vi "Subtask 3.vi"() -> ()   [LabVIEW 2016, in "LEGO-PMR.lvrbt"]
uses:
  LEGO-PMR.lvrbt
  <vilib>/NXT/Block Support/NXT_InputPort.ctl
  <vilib>/NXT/Block Support/NXT_OutputPort.ctl
  <vilib>/NXT/Dual Mode Library/Sensors/EV3_Ultrasonic_CM.vi
  <vilib>/NXT/NXTIO Xnodes/NXTIONodeSubVIs/NXTStopMotors.vi
  <vilib>/NXT/Dual Mode Library/Display/drawText.vi
  <vilib>/NXT/Dual Mode Library/Sensors/EV3_Color_Reflect.vi
  <vilib>/NXT/Dual Mode Library/Waits/Wait_Num(msec).vi
  <vilib>/NXT/NXTIO Xnodes/NXTIONodeSubVIs/NXTMoveMotors.vi
  <vilib>/NXT/Subs/LVHSConnector.ctl
  <vilib>/NXT/NXTIO Xnodes/AddressXNode/NXTIOAddress.xnode
  <vilib>/NXT/NXTIO Xnodes/NXTIOXNode/NXTIO.xnode
  <vilib>/NXT/LegoClasses/BrickReference/BrickReference.lvclass
panel:
  out "Arm Is Up":bool
  out "Output":string
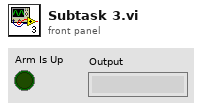
[diagram p1: front panel]
types:
  T1 = typedef "NXT_OutputPort.ctl" = u8
  T2 = typedef "NXT_InputPort.ctl" = u32
  T3 = typedef "LVHSConnector.ctl" = refnum<class "BrickReference.lvclass">
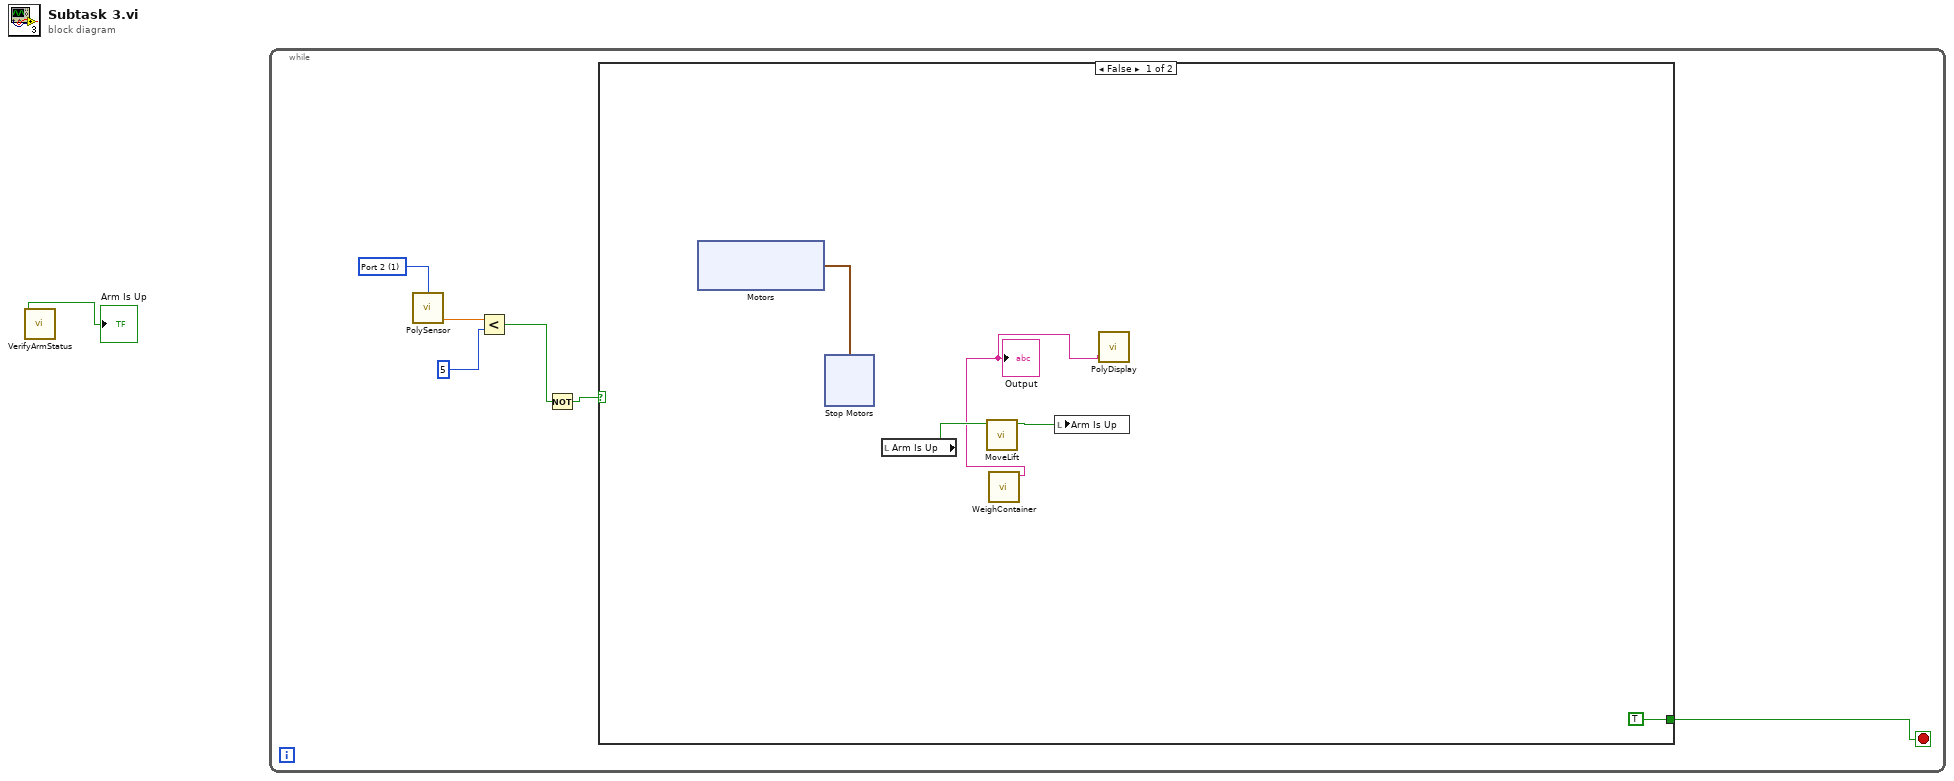
[diagram p0: block diagram]
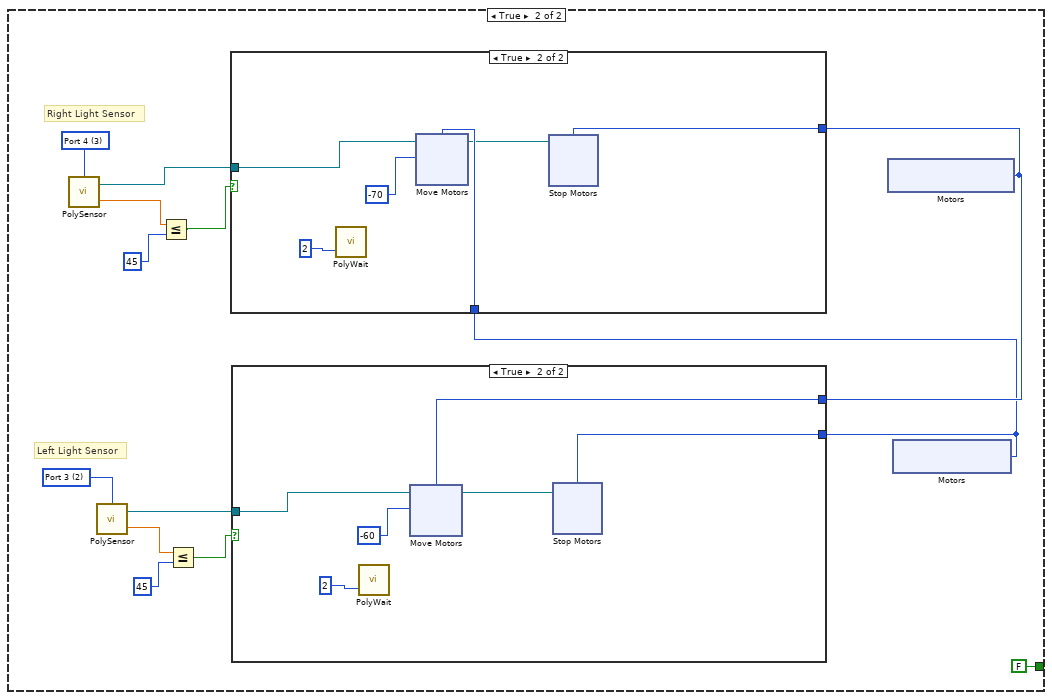
[diagram p2: hidden frame]
diagram:
  n1 = call "VerifyArmStatus.vi"() -> ("Is Arm Up?"=→"Arm Is Up":bool)  [unwired: 11 in]
  n2 = while {
    stop <- w2 stop-if-true
    w7 = T2 1 items=["Port 1", "Port 2", "Port 3", "Port 4"] ("Port (Port 1)")
    n3 = call-poly <vilib>:"PolySensor.vi"("Port (Port 1)"=w7) -> ("Centimeters"=w5:sgl)  [unwired: 2 in, 1 out]
    n4 = Less?(x=w5, y=5) -> (x < y?=w6:bool)
    n5 = Not(x=w6) -> (.not. x?=w3:bool)
    n6 = case shown="False" w3 {
      tunnel: [TRUE FALSE] -> w2
      frame False {
        n7 = xnode "Motors"() -> ("Motor"=w12:cluster{"Port":T1, "Port":T1})
        n8 = xnode "Stop Motors"("Motors"=w12) -> ()  [unwired: 1 in, 1 out]
        n9 = local read "Arm Is Up"() -> (w11:bool)
        n10 = call "MoveLift.vi"("Arm is Up?"=w11) -> ("Updated Bool"=w10:bool)  [unwired: 10 in]
        n11 = call "WeighContainer.vi"() -> ("Type"=w8:string)  [unwired: 10 in, 1 out]
        "Output" <- w8
        n12 = local write "Arm Is Up"(w10) -> ()
        n13 = call-poly <vilib>:"PolyDisplay.vi"("Text"=w8) -> ()  [unwired: 3 in, 1 out]
      }
      frame True {
        w30 = T2 3 items=["Port 1", "Port 2", "Port 3", "Port 4"] ("Port (Port 1)")
        w31 = T2 2 items=["Port 1", "Port 2", "Port 3", "Port 4"] ("Port (Port 1)")
        # "Left Light Sensor"
        # "Right Light Sensor"
        n14 = call-poly <vilib>:"PolySensor.vi"("Port (Port 1)"=w30) -> ("Scaled Value"=w24:sgl, "NXT/EV3"=w26:T3)  [unwired: 2 in]
        n15 = call-poly <vilib>:"PolySensor.vi"("Port (Port 1)"=w31) -> ("Scaled Value"=w22:sgl, "NXT/EV3"=w27:T3)  [unwired: 2 in]
        n16 = Less Or Equal?(x=w24, y=45) -> (x <= y?=w25:bool)
        n17 = Less Or Equal?(x=w22, y=45) -> (x <= y?=w20:bool)
        n18 = xnode "Motors"() -> ("Motor"=w29:T1)
        n19 = xnode "Motors"() -> ("Motor"=w28:T1)
        n20 = case shown="True" w25 {
          tunnel: w29 -> [_ w56]
          tunnel: w28 -> [_ w55]
          tunnel: w26 -> [_ w54]
          frame False {
          }
          frame True {
            n21 = call-poly <vilib>:"PolyWait.vi"("Time (100 msec)"=u32 2) -> ()  [unwired: 3 in, 1 out]
            n22 = xnode "Move Motors"("Power/Speed 1"=-70, "Motors"=w55, "NXT/EV3"=w54) -> ("NXT/EV3"=w53:T3)
            n23 = xnode "Stop Motors"("Motors"=w56, "NXT/EV3"=w53) -> ()  [unwired: 1 out]
          }
        }
        n24 = case shown="True" w20 {
          tunnel: w29 -> [_ w38]
          tunnel: w28 -> [_ w37]
          tunnel: w27 -> [_ w36]
          frame False {
          }
          frame True {
            n25 = call-poly <vilib>:"PolyWait.vi"("Time (100 msec)"=u32 2) -> ()  [unwired: 3 in, 1 out]
            n26 = xnode "Move Motors"("Power/Speed 1"=-60, "Motors"=w38, "NXT/EV3"=w36) -> ("NXT/EV3"=w35:T3)
            n27 = xnode "Stop Motors"("Motors"=w37, "NXT/EV3"=w35) -> ()  [unwired: 1 out]
          }
        }
      }
    }
  }
